vi "regUserEvent.vi"(8 "error in (no error)":errorcluster, 11 "tcpServer in":refnum<class "TcpServer.lvclass">) -> (0 "error out":errorcluster, 3 "tcpServer out":refnum<class "TcpServer.lvclass">)   [LabVIEW 2018, in "TcpServer.lvclass"]
doc: "Register User Events."
uses:
  TcpServer.lvclass
  typedef/ackTypeDef.ctl
  typedef/tcpPacketTypeDef.ctl
  typedef/userEventTypeDef.ctl
  typedef/eventTypeDef.ctl
  TcpServer.lvclass/TcpServer.ctl
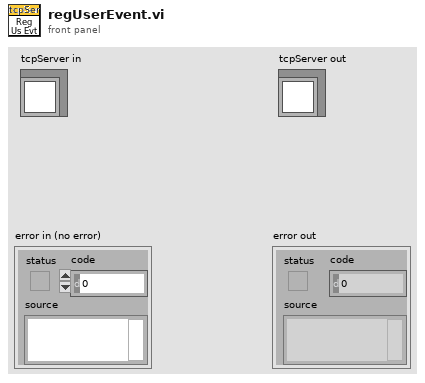
[diagram p1: front panel]
types:
  T1 = typedef "TcpServer.lvclass/tcpPacketTypeDef.ctl" = cluster{"packet":string, "firstPacket":bool, "firstConnection":bool}
  T2 = typedef "TcpServer.lvclass/eventTypeDef.ctl" = cluster{"evtName":string, "evtDetails":string}
  T3 = typedef "TcpServer.lvclass/userEventTypeDef.ctl" = cluster{"TcpServer":refnum<user-event>, "CmdRead":refnum<user-event>, "CmdWrite":refnum<user-event>, "MsgRead":refnum<user-event>, "MsgWrite":refnum<user-event>, "GenRead":refnum<user-event>, "GenWrite":refnum<user-event>}
  T4 = typedef "TcpServer.lvclass/ackTypeDef.ctl" = cluster{"tcpPacket":T1, "cmdStatus":string}
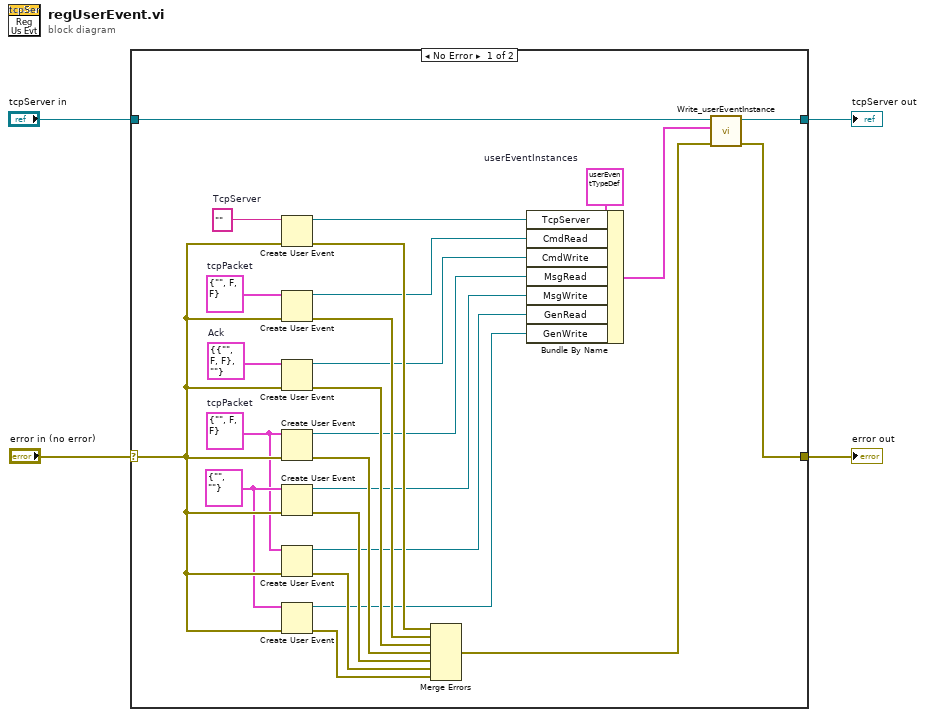
[diagram p0: block diagram]
diagram:
  n1 = case shown="No Error" "error in (no error)" {
    selector: "error in (no error)" -> [w13 w32]
    tunnel: [w28 w32] -> w3
    tunnel: [w29 w31] -> w1
    tunnel: "tcpServer in" -> [w30 w31]
    frame No Error {
      w7 = T1 {"packet"="", "firstPacket"=FALSE, "firstConnection"=FALSE}  # tcpPacket
      w10 = T2 {"evtName"="", "evtDetails"=""} ("Event")
      w15 = T1 {"packet"="", "firstPacket"=FALSE, "firstConnection"=FALSE}  # tcpPacket
      w18 = T3 {"TcpServer"=refnum, "CmdRead"=refnum, "CmdWrite"=refnum, "MsgRead"=refnum, "MsgWrite"=refnum, "GenRead"=refnum, "GenWrite"=refnum}  # userEventInstances
      w25 = ""  # TcpServer
      w26 = T4 {"tcpPacket"={"packet"="", "firstPacket"=FALSE, "firstConnection"=FALSE}, "cmdStatus"=""}  # Ack
      n2 = Create User Event(user event datatype=w25, error in=w13) -> (user event=w24:refnum<user-event>, error out=w23:errorcluster)
      n3 = Create User Event(user event datatype=w15, error in=w13) -> (user event=w17:refnum<user-event>, error out=w21:errorcluster)
      n4 = Create User Event(user event datatype=w26, error in=w13) -> (user event=w16:refnum<user-event>, error out=w20:errorcluster)
      n5 = Create User Event(user event datatype=w7, error in=w13) -> (user event=w6:refnum<user-event>, error out=w19:errorcluster)
      n6 = Create User Event(user event datatype=w10, error in=w13) -> (user event=w9:refnum<user-event>, error out=w14:errorcluster)
      n7 = Create User Event(user event datatype=w7, error in=w13) -> (user event=w5:refnum<user-event>, error out=w12:errorcluster)
      n8 = Create User Event(user event datatype=w10, error in=w13) -> (user event=w8:refnum<user-event>, error out=w11:errorcluster)
      n9 = Merge Errors(w23, w21, w20, w19, w14, w12, w11) -> (w22:errorcluster)
      n10 = Bundle By Name(cluster=w18, "TcpServer"=w24, "CmdRead"=w17, "CmdWrite"=w16, "MsgRead"=w6, "MsgWrite"=w9, "GenRead"=w5, "GenWrite"=w8) -> (w27:T3)
      n11 = call "Write_userEventInstance.vi"("error in (no error)"=w22, "UserEvents"=w27, "tcpServer in"=w30) -> ("error out"=w28:errorcluster, "tcpServer out"=w29:refnum<class "TcpServer.lvclass">)  [unwired: 7 in]
    }
    frame Error {
    }
  }
  "error out" <- w3
  "tcpServer out" <- w1
